vi "setUserEvent.vi"(8 "error in (no error)":errorcluster, 11 "CoolDisplay in":refnum<class "CoolDisplay.lvclass">) -> (0 "error out":errorcluster, 3 "CoolDisplay out":refnum<class "CoolDisplay.lvclass">)   [LabVIEW 2018, in "CoolDisplay.lvclass"]
uses:
  CoolDisplay.lvclass
  Observer/Observer.lvclass
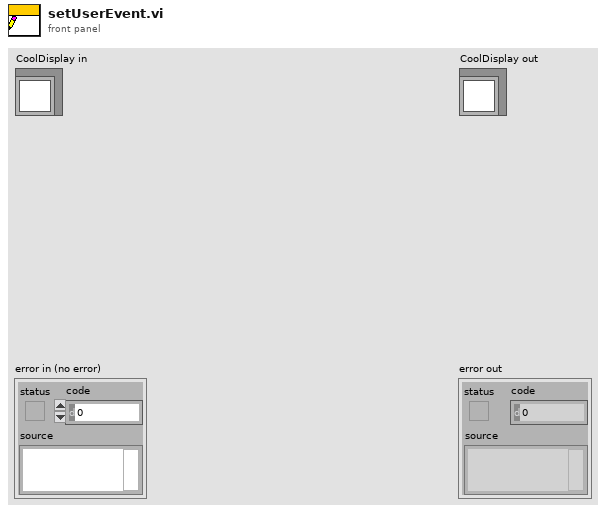
[diagram p1: front panel]
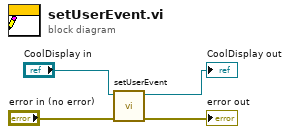
[diagram p0: block diagram]
diagram:
  n1 = call-parent "setUserEvent.vi"("error in (no error)"="error in (no error)", "Observer in"="CoolDisplay in") -> ("error out"=→"error out":errorcluster, "Observer out"=→"CoolDisplay out":refnum<class "CoolDisplay.lvclass">)  [unwired: 8 in]
